vi "Output Example.vi"(8 "error in":errorcluster, 11 "UDP in":refnum<class "UDP.lvclass">) -> (0 "error out":errorcluster, 3 "UDP out":refnum<class "UDP.lvclass">)   [LabVIEW 2020, in "Plugin Instrument Driver.lvlib" / "UDP.lvclass"]
doc: "Initialize connection, Set Configre & Close the connection"
uses:
  UDP.lvclass
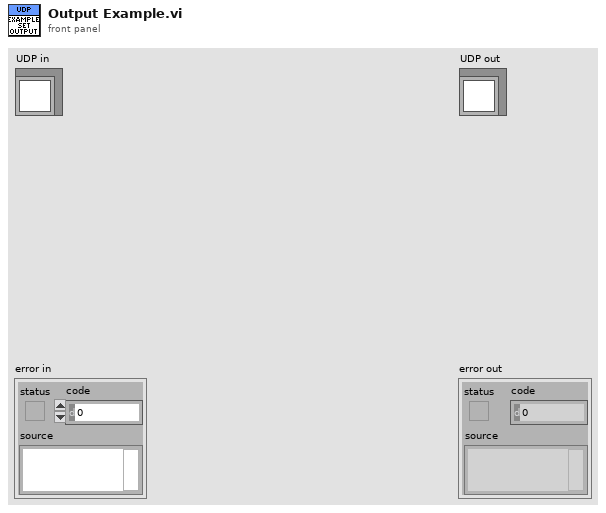
[diagram p1: front panel]
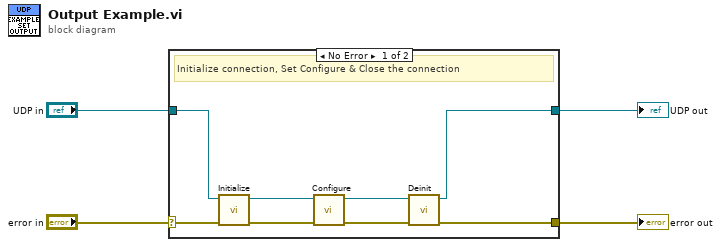
[diagram p0: block diagram]
diagram:
  n1 = case shown="No Error" "error in" {
    selector: "error in" -> [w6 w14]
    tunnel: [w5 w14] -> w3
    tunnel: [w7 w13] -> w1
    tunnel: "UDP in" -> [w8 w13]
    frame No Error {
      # "Initialize connection, Set Configure & Close the connection"
      n2 = call-dynamic "Initialize.vi"("error in"=w6, "UDP in"=w8) -> ("error out"=w11:errorcluster, "UDP out"=w12:refnum<class "UDP.lvclass">)  [unwired: 8 in]
      n3 = call-dynamic "Configure.vi"("error in"=w11, "UDP in"=w12) -> ("error out"=w9:errorcluster, "UDP out"=w10:refnum<class "UDP.lvclass">)  [unwired: 8 in]
      n4 = call-dynamic "Deinit.vi"("error in"=w9, "UDP in"=w10) -> ("error out"=w5:errorcluster, "UDP out"=w7:refnum<class "UDP.lvclass">)  [unwired: 8 in]
    }
    frame Error {
    }
  }
  "error out" <- w3
  "UDP out" <- w1
